vi "DC_Daemont.vi"() -> ()   [LabVIEW 2013, in "double click.lvlib"]
uses:
  double click.lvlib
panel:
  in  "Path":path
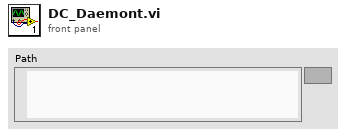
[diagram p1: front panel]
types:
  T1 = enum32{"Invalid", "Standard", "Closed", "Hidden", "Minimized", "Maximized"}
  T2 = cluster{"App Dir":path, "App Kind":enum32{"invalid app kind", "Development System", "Run Time System", "Student Edition", "Embedded LabVIEW", "Evaluation", "Custom"}, "App Ref":refnum<vi>, "Client":string, "Client Port":u16, "Handler VI ref":refnum<vi>, "Timeout timer":u32}
  T3 = enum32{"Bad", "Idle", "Run top level", "Running"}
  T4 = enum32{"invalid app kind", "Development System", "Run Time System", "Student Edition", "Embedded LabVIEW", "Evaluation", "Custom"}
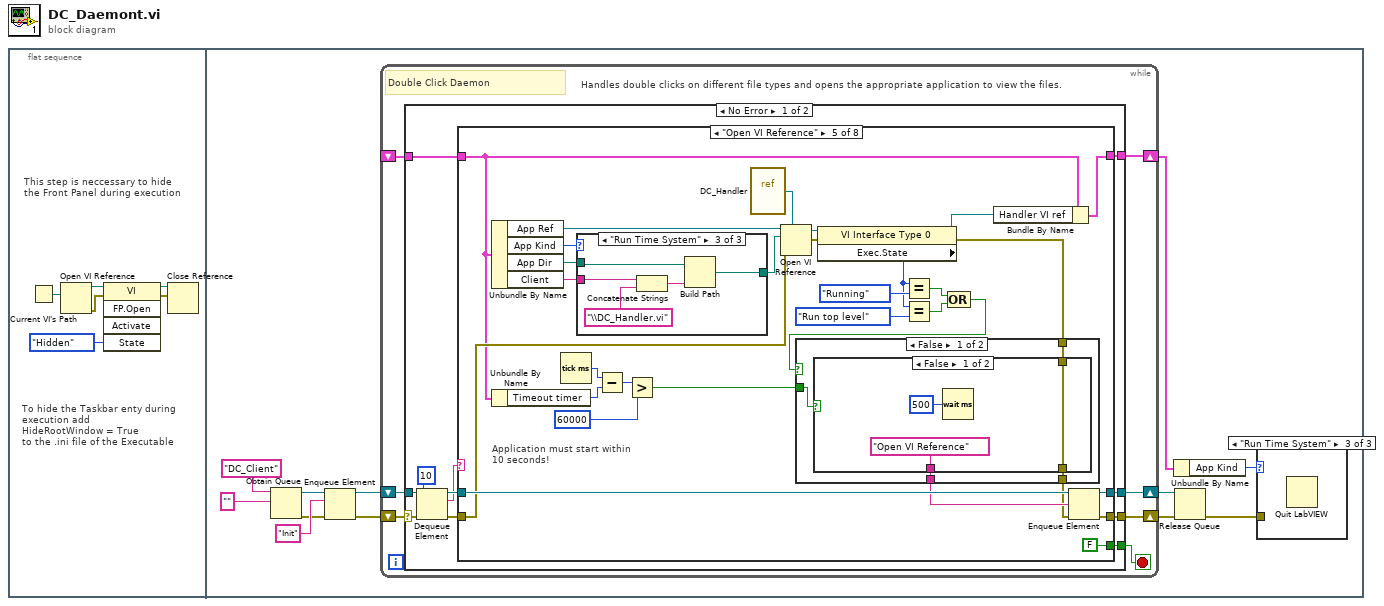
[diagram p0: block diagram]
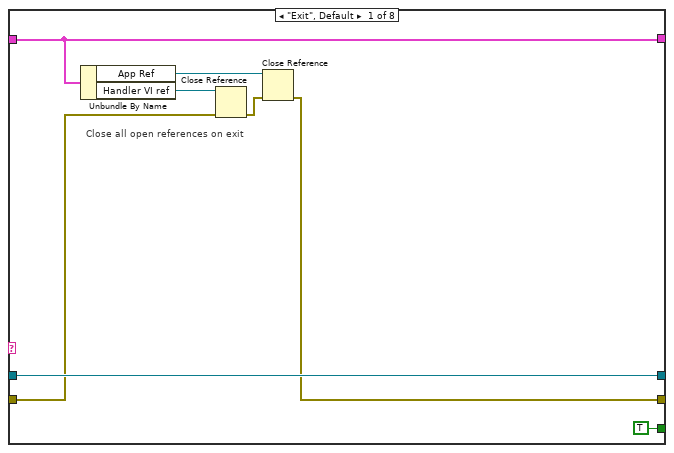
[diagram p4: hidden frame]
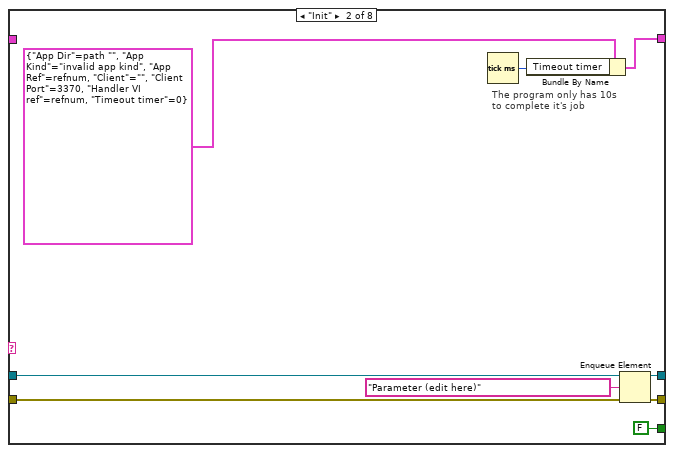
[diagram p5: hidden frame]
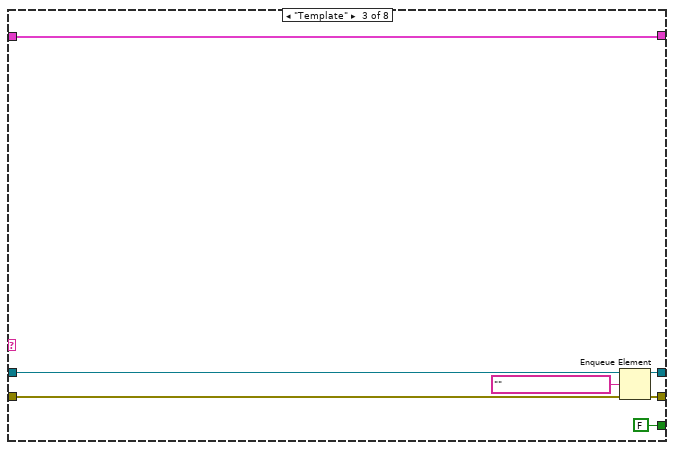
[diagram p6: hidden frame]
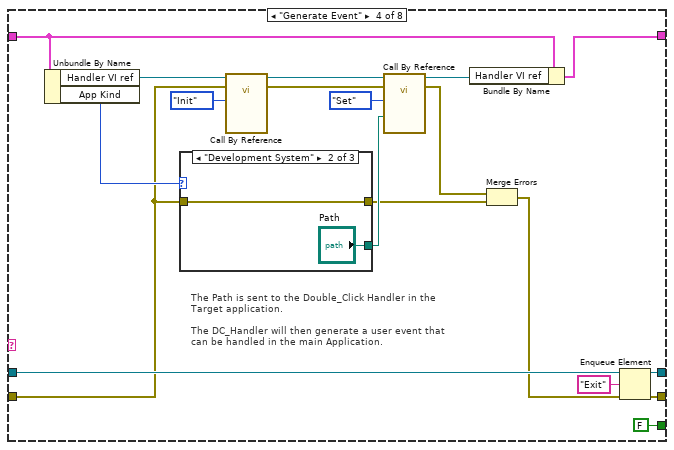
[diagram p7: hidden frame]
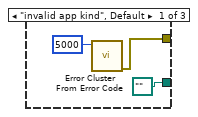
[diagram p8: hidden frame]
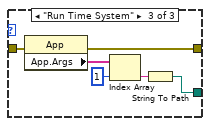
[diagram p9: hidden frame]
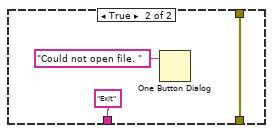
[diagram p10: hidden frame]
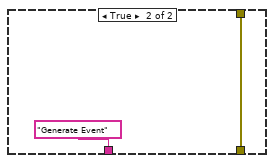
[diagram p11: hidden frame]
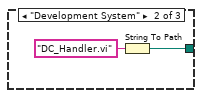
[diagram p13: hidden frame]
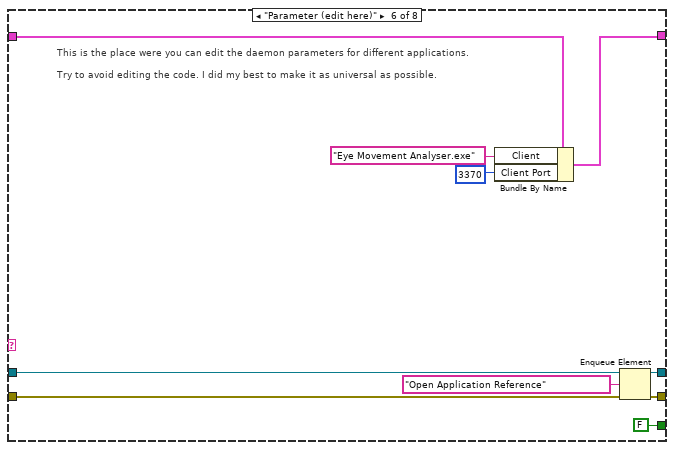
[diagram p14: hidden frame]
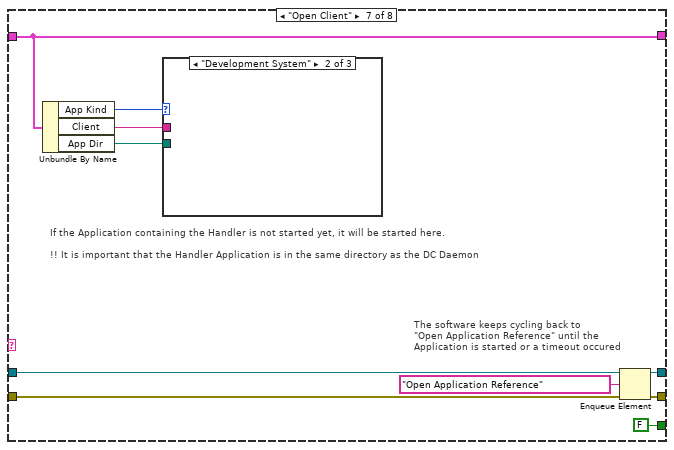
[diagram p15: hidden frame]
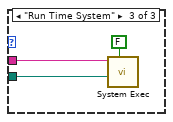
[diagram p17: hidden frame]
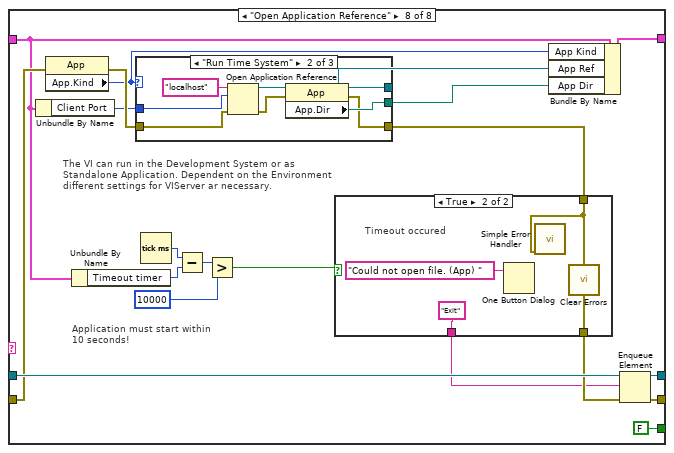
[diagram p18: hidden frame]
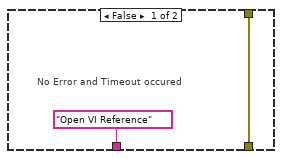
[diagram p19: hidden frame]
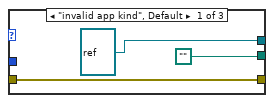
[diagram p20: hidden frame]
diagram:
  n1 = flat-sequence {
    frame #0 {
      # "To hide the Taskbar enty during\nexecution add\nHideRootWindow = True\nto the .ini file of the Executable"
      # "This step is neccessary to hide\nthe Front Panel during execution"
      n2 = Current VI's Path() -> (path=w6:path)
      n3 = Open VI Reference(vi path=w6) -> (vi reference=w5:refnum<vi>, error out=w4:errorcluster)  [unwired: 5 in]
      n4 = invoke class="VI" method="FP.Open"(reference=w5, error in=w4, "State"=T1."Hidden") -> (reference out=w1:refnum<vi>, error out=w2:errorcluster)  [unwired: 2 in, 3 out]
      n5 = Close Reference(reference=w1, error in (no error)=w2) -> ()  [unwired: 1 out]
    }
    frame #1 {
      n6 = Obtain Queue(name (unnamed)="DC_Client", element data type="") -> (queue out=w16:refnum<queue>, error out=w12:errorcluster)  [unwired: 3 in, 1 out]
      n7 = Enqueue Element(queue=w16, element="Init", error in (no error)=w12) -> (queue out=w14:refnum<queue>, error out=w13:errorcluster)  [unwired: 1 in, 1 out]
      n8 = while {
        shift-right: [w23] -> w10
        shift-left: w13 -> [w24]
        shift-right: [w21] -> w11
        shift-left: w14 -> [w25]
        shift-right: [w20] -> w9
        shift-left: _ -> [w19]
        stop <- w22 stop-if-true
        # "Handles double clicks on different file types and opens the appropriate application to view the files."
        # "Double Click Daemon"
        n9 = case shown="No Error" w24 {
          selector: w24 -> [w35 w204]
          tunnel: w25 -> [w36 w205]
          tunnel: [w34 w206] -> w23
          tunnel: [w32 FALSE] -> w22
          tunnel: [w31 w207] -> w21
          tunnel: [w27 w210] -> w20
          tunnel: w19 -> [w26 w210]
          frame No Error {
            n10 = Dequeue Element(queue=w36, timeout in ms (-1)=10, error in (no error)=w35) -> (queue out=w30:refnum<queue>, element=w29:string, error out=w33:errorcluster)  [unwired: 1 out]
            n11 = case shown="\"Open VI Reference\"" w29 {
              tunnel: [w37 w52 w59 w78 w119 w148 w158 w181] -> w34
              tunnel: w33 -> [w38 w50 w57 w61 w106 w146 w156 w176]
              tunnel: [TRUE FALSE FALSE FALSE FALSE FALSE FALSE FALSE] -> w32
              tunnel: [w44 w51 w58 w77 w118 w147 w157 w180] -> w31
              tunnel: w30 -> [w44 w49 w56 w76 w117 w145 w155 w179]
              tunnel: [w42 w46 w54 w70 w110 w140 w153 w178] -> w27
              tunnel: w26 -> [w42 _ w54 w71 w100 w141 w153 w168]
              frame "Exit", Default {
                # "Close all open references on exit"
                n12 = Unbundle By Name(w42) -> ("App Ref"=w39:refnum<vi>, "Handler VI ref"=w40:refnum<vi>)
                n13 = Close Reference(reference=w40, error in (no error)=w38) -> (error out=w41:errorcluster)
                n14 = Close Reference(reference=w39, error in (no error)=w41) -> (error out=w37:errorcluster)
              }
              frame "Init" {
                # "The program only has 10s \nto complete it's job"
                n15 = Tick Count (ms)() -> (millisecond timer value=w45:u32)
                n16 = Bundle By Name(cluster=T2 {"App Dir"=path "", "App Kind"=enum."invalid app kind", "App Ref"=refnum, "Client"="", "Client Port"=3370, "Handler VI ref"=refnum, "Timeout timer"=0}, "Timeout timer"=w45) -> (w46:T2)
                n17 = Enqueue Element(queue=w49, element="Parameter (edit here)", error in (no error)=w50) -> (queue out=w51:refnum<queue>, error out=w52:errorcluster)  [unwired: 1 in, 1 out]
              }
              frame "Template" {
                n18 = Enqueue Element(queue=w56, element="", error in (no error)=w57) -> (queue out=w58:refnum<queue>, error out=w59:errorcluster)  [unwired: 1 in, 1 out]
              }
              frame "Generate Event" {
                # "The Path is sent to the Double_Click Handler in the \nTarget application. \n\nThe DC_Handler will then generate a user event that\ncan be handled in the main Application."
                n19 = Unbundle By Name(w71) -> ("Handler VI ref"=w69:refnum<vi>, "App Kind"=w65:T4)
                n20 = case shown="\"Development System\"" w65 {
                  tunnel: [path "" ("Path") "Path" w87] -> w73
                  tunnel: w61 -> [_ w84 w86]
                  tunnel: [w82 w84 w85] -> w64
                  frame "invalid app kind", Default {
                    n21 = call <vilib>:"Error Cluster From Error Code.vi"("error code (0)"=5000) -> ("error out"=w82:errorcluster)  [unwired: 8 in]
                  }
                  frame "Development System" {
                  }
                  frame "Run Time System" {
                    n22 = property class="App"(error in=w86) -> (error out=w85:errorcluster, "App.Args"=w89:string[])  [unwired: 1 in, 1 out]
                    n23 = Index Array(array=w89, index=1) -> (element=w88:string)
                    n24 = String To Path(string=w88) -> (path=w87:path)
                  }
                }
                n25 = call-by-ref "?"(reference=w69, error in=w61, "Operation"=enum16{"Init", "Set"}."Init") -> (reference out=w68:refnum<vi>, error out=w66:errorcluster)  [unwired: 10 in, 1 out]
                n26 = call-by-ref "?"(reference=w68, error in=w66, "file"=w73, "Operation"=enum16{"Init", "Set"}."Set") -> (reference out=w72:refnum<vi>, error out=w63:errorcluster)  [unwired: 9 in, 1 out]
                n27 = Bundle By Name(cluster=w71, "Handler VI ref"=w72) -> (w70:T2)
                n28 = Merge Errors(w63, w64) -> (w62:errorcluster)
                n29 = Enqueue Element(queue=w76, element="Exit", error in (no error)=w62) -> (queue out=w77:refnum<queue>, error out=w78:errorcluster)  [unwired: 1 in, 1 out]
              }
              frame "Open VI Reference" {
                # "Application must start within\n10 seconds!"
                n30 = Unbundle By Name(w100) -> ("App Ref"=w116:refnum<vi>, "App Kind"=w114:T4, "App Dir"=w113:path, "Client"=w112:string)
                n31 = Unbundle By Name(w100) -> ("Timeout timer"=w98:u32)
                n32 = Tick Count (ms)() -> (millisecond timer value=w99:u32)
                n33 = case shown="\"Run Time System\"" w114 {
                  tunnel: w113 -> [_ _ w136]
                  tunnel: w112 -> [_ _ w139]
                  tunnel: [_ w134 w135] -> w111
                  frame "invalid app kind", Default {
                  }
                  frame "Development System" {
                    n34 = String To Path(string="DC_Handler.vi") -> (path=w134:path)
                  }
                  frame "Run Time System" {
                    n35 = Concatenate Strings(w139, "\\DC_Handler.vi" ("string")) -> (w137:string)
                    n36 = Build Path(base path=w136, name or relative path=w137) -> (appended path=w135:path)
                  }
                }
                n37 = Subtract(x=w99, y=w98) -> (x-y=w97:u32)
                n38 = Greater?(x=w97, y=u32 60000) -> (0:w92:bool)
                n39 = vi-ref "DC_Handler.vi"() -> (w115:refnum<vi>)
                n40 = Open VI Reference(type specifier VI Refnum (for type only)=w115, application reference (local)=w116, vi path=w111, error in (no error)=w106) -> (vi reference=w109:refnum<vi>, error out=w107:errorcluster)  [unwired: 2 in]
                n41 = property class="VI Interface Type 0"(reference=w109, error in=w107) -> (reference out=w108:refnum<vi>, error out=w94:errorcluster, "Exec.State"=w104:T3)
                n42 = Equal?(x=w104, y=T3."Running") -> (x = y?=w102:bool)
                n43 = Equal?(x=w104, y=T3."Run top level") -> (x = y?=w101:bool)
                n44 = Compound Arithmetic op=OR(w102, w101) -> (w91:bool)
                n45 = case shown="False" w91 {
                  tunnel: w92 -> [w124 _]
                  tunnel: [w123 "Generate Event" ("element")] -> w95
                  tunnel: w94 -> [w122 w131]
                  tunnel: [w121 w131] -> w93
                  frame False {
                    n46 = case shown="False" w124 {
                      tunnel: ["Open VI Reference" ("element") "Exit" ("element")] -> w123
                      tunnel: w122 -> [w126 w128]
                      tunnel: [w126 w128] -> w121
                      frame False {
                        n47 = Wait (ms)(milliseconds to wait=u32 500) -> ()  [unwired: 1 out]
                      }
                      frame True {
                        n48 = One Button Dialog(message="Could not open file. ") -> ()  [unwired: 1 in, 1 out]
                      }
                    }
                  }
                  frame True {
                  }
                }
                n49 = Bundle By Name(cluster=w100, "Handler VI ref"=w108) -> (w110:T2)
                n50 = Enqueue Element(queue=w117, element=w95, error in (no error)=w93) -> (queue out=w118:refnum<queue>, error out=w119:errorcluster)  [unwired: 1 in, 1 out]
              }
              frame "Parameter (edit here)" {
                # "This is the place were you can edit the daemon parameters for different applications.\n\nTry to avoid editing the code. I did my best to make it as universal as possible."
                n51 = Bundle By Name(cluster=w141, "Client"="Eye Movement Analyser.exe", "Client Port"=u16 3370) -> (w140:T2)
                n52 = Enqueue Element(queue=w145, element="Open Application Reference", error in (no error)=w146) -> (queue out=w147:refnum<queue>, error out=w148:errorcluster)  [unwired: 1 in, 1 out]
              }
              frame "Open Client" {
                # "The software keeps cycling back to \n\"Open Application Reference\" until the\nApplication is started or a timeout occured"
                # "If the Application containing the Handler is not started yet, it will be started here. \n\n!! It is important that the Handler Application is in the same directory as the DC Daemon"
                n53 = Unbundle By Name(w153) -> ("App Kind"=w152:T4, "Client"=w150:string, "App Dir"=w151:path)
                n54 = case shown="\"Development System\"" w152 {
                  tunnel: w151 -> [_ _ w161]
                  tunnel: w150 -> [_ _ w160]
                  frame "invalid app kind", Default {
                  }
                  frame "Development System" {
                  }
                  frame "Run Time System" {
                    n55 = call <vilib>:"System Exec.vi"("wait until completion? (T)"=FALSE, "working directory"=w161, "command line"=w160) -> ()  [unwired: 5 in, 4 out]
                  }
                }
                n56 = Enqueue Element(queue=w155, element="Open Application Reference", error in (no error)=w156) -> (queue out=w157:refnum<queue>, error out=w158:errorcluster)  [unwired: 1 in, 1 out]
              }
              frame "Open Application Reference" {
                # "Application must start within\n10 seconds!"
                # "The VI can run in the Development System or as\nStandalone Application. Dependent on the Environment\ndifferent settings for VIServer ar necessary."
                n57 = Unbundle By Name(w168) -> ("Client Port"=w173:u16)
                n58 = property class="App"(error in=w176) -> (error out=w177:errorcluster, "App.Kind"=w175:T4)  [unwired: 1 in, 1 out]
                n59 = Unbundle By Name(w168) -> ("Timeout timer"=w171:u32)
                n60 = case shown="\"Run Time System\"" w175 {
                  tunnel: [refnum<vi> refnum ("application reference") w195 w203] -> w163
                  tunnel: [path "" w194 w202] -> w174
                  tunnel: w177 -> [w189 w198 w201]
                  tunnel: [w189 w192 w200] -> w166
                  tunnel: w173 -> [_ w197 _]
                  frame "invalid app kind", Default {
                  }
                  frame "Run Time System" {
                    n61 = Open Application Reference(8:w198, 10:w197, 11:"localhost" ("machine name (\"\":  open local reference)")) -> (0:w193:errorcluster, 3:w196:refnum<vi>)  [unwired: 1 in]
                    n62 = property class="App"(reference=w196, error in=w193) -> (reference out=w195:refnum<vi>, error out=w192:errorcluster, "App.Dir"=w194:path)
                  }
                  frame "Development System" {
                    n63 = Open Application Reference(8:w201) -> (0:w200:errorcluster, 3:w203:refnum<vi>)  [unwired: 3 in]
                    n64 = Current VI's Path() -> (path=w202:path)
                  }
                }
                n65 = Tick Count (ms)() -> (millisecond timer value=w172:u32)
                n66 = Subtract(x=w172, y=w171) -> (x-y=w170:u32)
                n67 = Greater?(x=w170, y=u32 10000) -> (0:w167:bool)
                n68 = case shown="True" w167 {
                  tunnel: ["Open VI Reference" ("element") "Exit" ("element")] -> w164
                  tunnel: w166 -> [w184 w185]
                  tunnel: [w184 w186] -> w165
                  frame False {
                    # "No Error and Timeout occured"
                  }
                  frame True {
                    # "Timeout occured"
                    n69 = One Button Dialog(message="Could not open file. (App) ") -> ()  [unwired: 1 in, 1 out]
                    n70 = call <vilib>:"Simple Error Handler.vi"("error in (no error)"=w185) -> ()  [unwired: 4 in, 5 out]
                    n71 = call <vilib>:"Clear Errors.vi"("error in (no error)"=w185) -> ("error out"=w186:errorcluster)  [unwired: 6 in]
                  }
                }
                n72 = Bundle By Name(cluster=w168, "App Kind"=w175, "App Ref"=w163, "App Dir"=w174) -> (w178:T2)
                n73 = Enqueue Element(queue=w179, element=w164, error in (no error)=w165) -> (queue out=w180:refnum<queue>, error out=w181:errorcluster)  [unwired: 1 in, 1 out]
              }
            }
          }
          frame Error {
            n74 = Unbundle By Name(w204) -> ("code"=w208:i32)
            n75 = case shown="63" w208 {
              tunnel: [w216 w227 w234] -> w207
              tunnel: [w215 w226 w233] -> w206
              tunnel: w205 -> [w214 w225 w232]
              tunnel: w204 -> [w211 _ _]
              frame 0, Default {
                # "Not handled error"
                n76 = call <vilib>:"Simple Error Handler.vi"("error in (no error)"=w211) -> ("error out"=w212:errorcluster)  [unwired: 4 in, 4 out]
                n77 = call <vilib>:"Clear Errors.vi"("error in (no error)"=w212) -> ("error out"=w213:errorcluster)  [unwired: 6 in]
                n78 = Flush Queue(queue=w214, error in (no error)=w213) -> (queue out=w218:refnum<queue>, error out=w217:errorcluster)  [unwired: 1 out]
                n79 = Enqueue Element(queue=w218, element="Exit", error in (no error)=w217) -> (queue out=w216:refnum<queue>, error out=w215:errorcluster)  [unwired: 1 in, 1 out]
              }
              frame 63 {
                # "Code 63 occurs if the VIServer Client (e.g. EMA2010 Main program) is not runing."
                n80 = First Call?() -> (First Call?: T/F=w223:bool)
                n81 = Select(t="Open Client" ("element"), s=w223, f="Open Application Reference" ("element")) -> (s? t:f=w220:string)
                n82 = call <vilib>:"Clear Errors.vi"() -> ("error out"=w224:errorcluster)  [unwired: 7 in]
                n83 = Flush Queue(queue=w225, error in (no error)=w224) -> (queue out=w229:refnum<queue>, error out=w228:errorcluster)  [unwired: 1 out]
                n84 = Enqueue Element(queue=w229, element=w220, error in (no error)=w228) -> (queue out=w227:refnum<queue>, error out=w226:errorcluster)  [unwired: 1 in, 1 out]
              }
              frame 1025 {
                # "Code 1025 occurs during Check Client Status, until Client is running."
                n85 = call <vilib>:"Clear Errors.vi"() -> ("error out"=w231:errorcluster)  [unwired: 7 in]
                n86 = Flush Queue(queue=w232, error in (no error)=w231) -> (queue out=w236:refnum<queue>, error out=w235:errorcluster)  [unwired: 1 out]
                n87 = Wait (ms)(milliseconds to wait=u32 200) -> ()  [unwired: 1 out]
                n88 = Enqueue Element(queue=w236, element="Open VI Reference", error in (no error)=w235) -> (queue out=w234:refnum<queue>, error out=w233:errorcluster)  [unwired: 1 in, 1 out]
              }
            }
          }
        }
      }
      n89 = Unbundle By Name(w9) -> ("App Kind"=w8:T4)
      n90 = Release Queue(queue=w11, error in (no error)=w10) -> (error out=w7:errorcluster)  [unwired: 1 in, 2 out]
      n91 = case shown="\"Run Time System\"" w8 {
        tunnel: w7 -> [_ _ _]
        frame "invalid app kind", Default {
        }
        frame "Development System" {
        }
        frame "Run Time System" {
          n92 = Quit LabVIEW() -> ()  [unwired: 1 in]
        }
      }
    }
  }
